vi "Concentration Calculation.vi"(8 "error in (no error)":errorcluster, 9 "Total Volume (µL)":dbl, 10 "Required Concentration\n(M)":dbl[](array[numeric]), 11 "Reservoir Concentrations\n(M)":dbl[](array[numeric])) -> (0 "error out":errorcluster, 2 "Solvent Volume (µL)":dbl, 3 "Reagent Volume (µL)":dbl[](array[numeric]))   [LabVIEW 2020]
uses:
  <vilib>/Utility/error.llb/Error Cluster From Error Code.vi
  <vilib>/ErrorRing/Error Ring.xnode
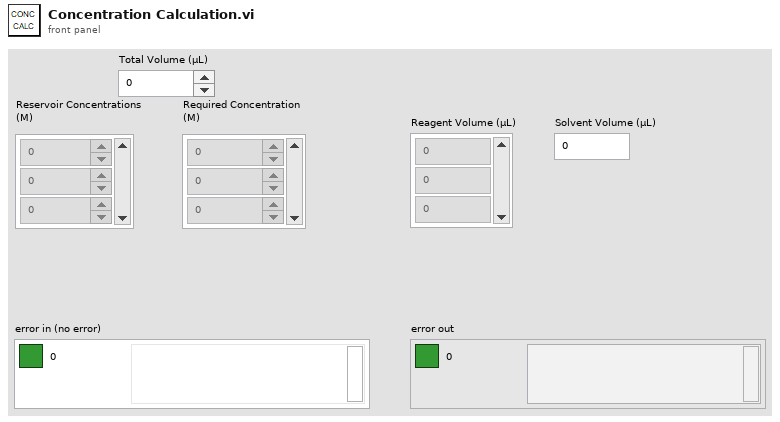
[diagram p1: front panel]
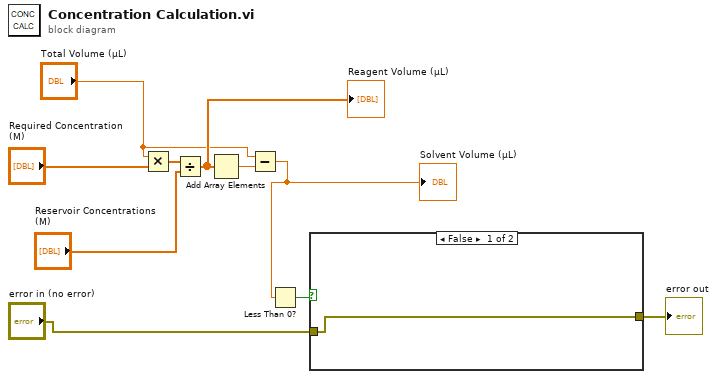
[diagram p0: block diagram]
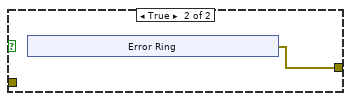
[diagram p2: hidden frame]
diagram:
  n1 = Multiply(x="Total Volume (µL)", y="Required Concentration\n(M)") -> (x*y=w8:dbl[])
  n2 = Divide(x=w8, y="Reservoir Concentrations\n(M)") -> (x/y=w7:dbl[])
  "Reagent Volume (µL)" <- w7
  n3 = Add Array Elements(numeric array=w7) -> (sum=w5:dbl)
  n4 = Subtract(x="Total Volume (µL)", y=w5) -> (x-y=w3:dbl)
  "Solvent Volume (µL)" <- w3
  n5 = Less Than 0?(x=w3) -> (x < 0?=w4:bool)
  n6 = case shown="False" w4 {
    tunnel: "error in (no error)" -> [w11 _]
    tunnel: [w11 w12] -> w1
    frame False {
    }
    frame True {
      n7 = xnode "Error Ring"() -> ("error out"=w12:errorcluster)
    }
  }
  "error out" <- w1
